vi "test_delay_line_ASIC.vi"(4 "Voltages comprobation":dbl[](array[numeric])=[0.05, 0.06, 0.07, 0.08, 0.09, 0.1, 0.2, 0.3, 0.4, 0.5, 0.6, 0.7, 0.8, 0.9, 1.0], 8 "error in":errorcluster, 9 "Cycles Burst":i32=10000, 11 "Instrument VISA in":T1={"AWG VISA"="generadorpulsos", "Oscilloscope  VISA "="Oscilloscope", "Integration Board IP"="172.16.7.43", "connection ID"=refnum, "report out"=refnum, "report file path"=path "D:/CTA/Data_test/ASIC/delay_line_test"}) -> (0 "error out":errorcluster, 3 "Instrument VISA out":T1={"AWG VISA"="81160A", "Oscilloscope  VISA "="DSO80204B", "Integration Board IP"="172.16.7.43", "connection ID"=refnum, "report out"=refnum, "report file path"=path "D:/CTA/LevelTriggerBoardTest/TestsData/sumtrigger_delay/dataruben"})   [LabVIEW 2009]
uses:
  <vilib>/Utility/NIReport.llb/NI_report.lvclass
  <vilib>/Utility/NIReport.llb/HTML/NI_HTML.lvclass
  <instrlib>/Agilent 8000 Series/Public/Configure/Configure Trigger (Edge).vi
  <instrlib>/Agilent 81150/Agilent 81150.lvlib
  <instrlib>/Agilent 8000 Series/Agilent 8000 Series.lvlib
panel:
  out "Waveform Graph 2":dbl[](graph)
  out "Waveform Graph":dbl[](graph)
  out "XY Graph":cluster{"Y":dbl[], "Y":dbl[]}[](graph)
  out "data read value 18":u32
  out "data out serial 18":string
  out "Data to send hex 18":string
  out "Delay value 2":u16(ring) items=["0", "0.25ns", "0.5ns", "0.75ns", "1ns", "1.25ns", "1.5ns", "1.75ns", "2ns", "2.25ns", "2.5ns", "2.75ns", "3ns", "3.25ns", "3.5ns", "3.75ns", "4ns", "4.25ns", "4.5ns", "4.75ns", "5ns", "5.25ns", "5.5ns", "5.75ns", "2ns_b", "2.25ns_b", "2.5ns_b", "2.75ns_b", "3ns_b", "3.25ns_b", "3.5ns_b", "3.75ns_b", ""]
  out "Id out":i32
  out "Value hex":u32
  in  "Oscilloscope?":bool
  in  "Delay Time (s)":dbl=0.5
  in  "channel":i32
  out "report file path":path
  out "Data output":dbl[][](array[numeric])=[[0.05, 0.0, 0.0, 9.0, 0.0, 0.0, 0.0, 0.0, 0.0, 0.0, 0.0, 0.0, 0.0, 0.0, 0.0, 0.0, 0.036000000000000004, 0.0]]
  out "bucle time":u32=10690
  out "read buffer 3":string
  out "appended array":dbl[](array[numeric])
  out "Numeric":i32=79625954
  in  "Save NOW!":bool
  in  "End 2":bool
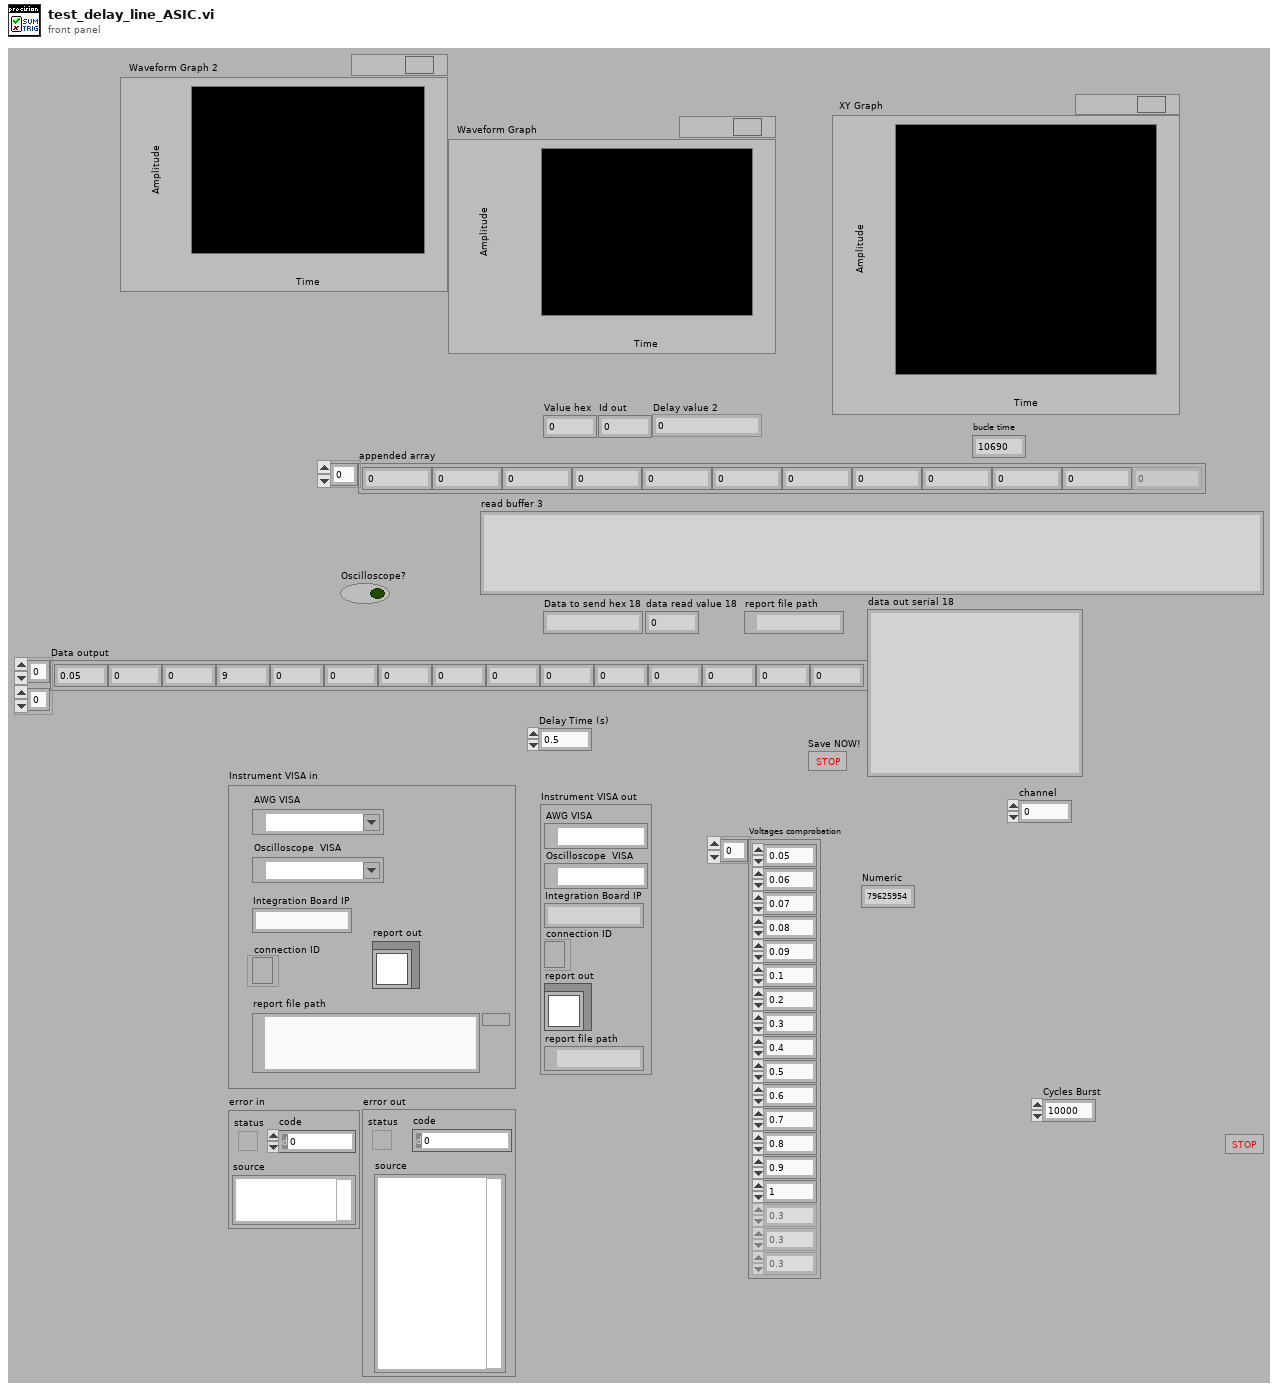
[diagram p1: front panel]
types:
  T1 = cluster{"AWG VISA":refnum<visa-resource-name>, "Oscilloscope  VISA ":refnum<visa-resource-name>, "Integration Board IP":string, "connection ID":refnum<k5>, "report out":refnum<class "NI_report.lvclass">, "report file path":path}
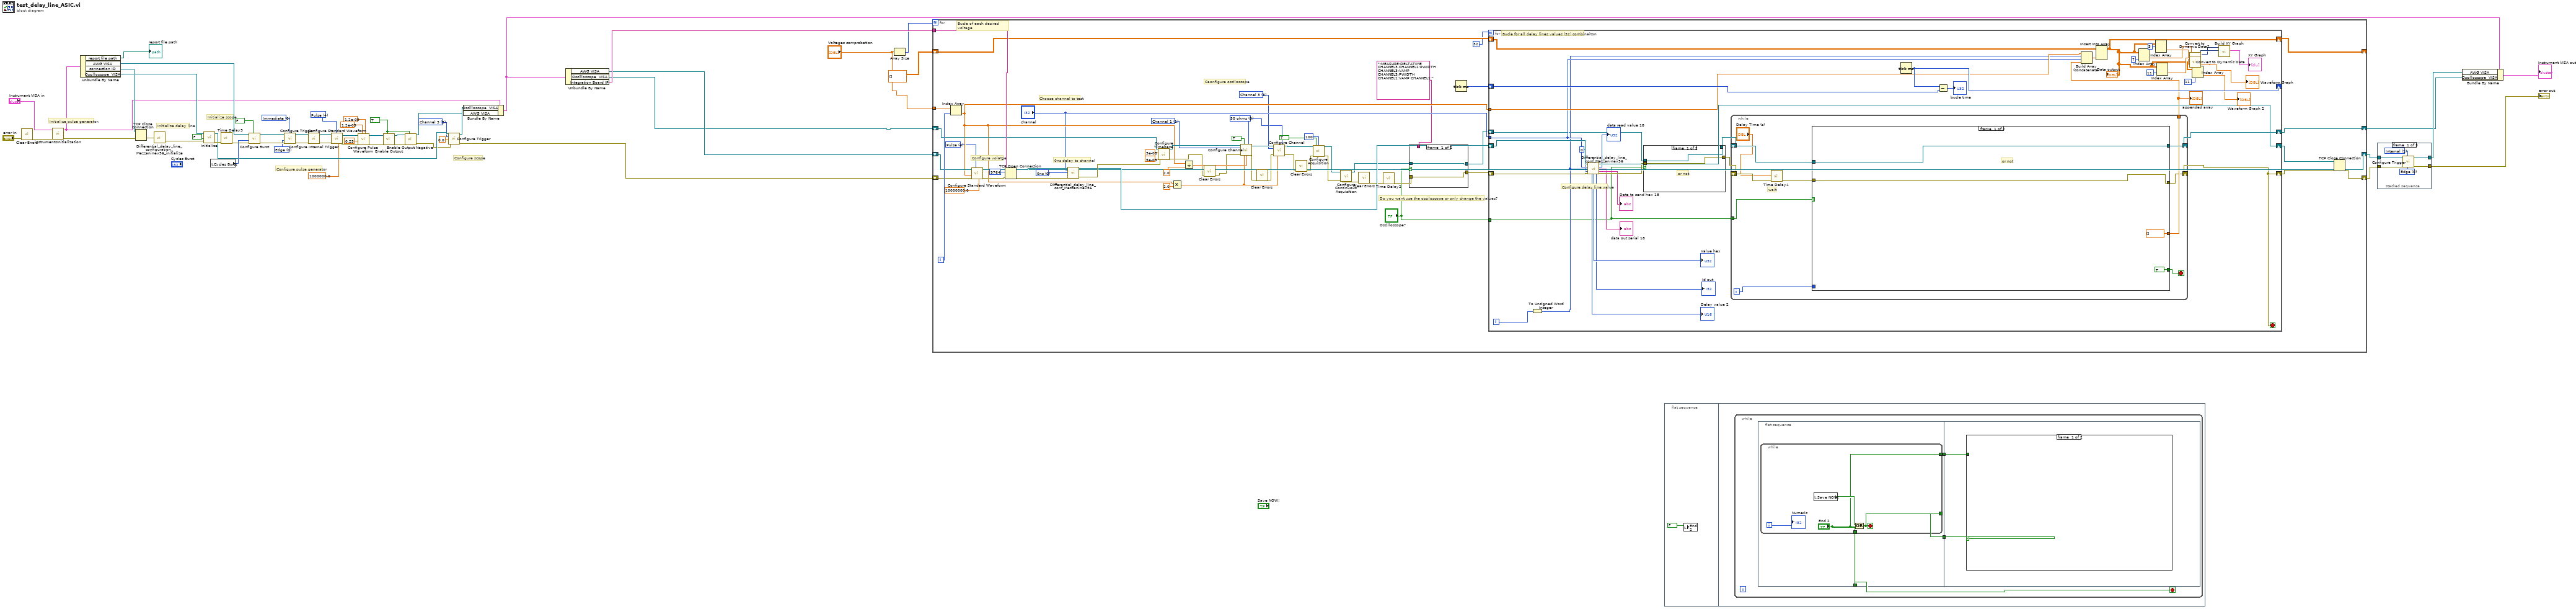
[diagram p0: block diagram]
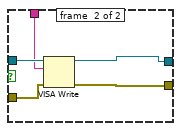
[diagram p2: hidden frame]
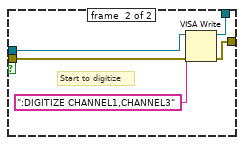
[diagram p3: hidden frame]
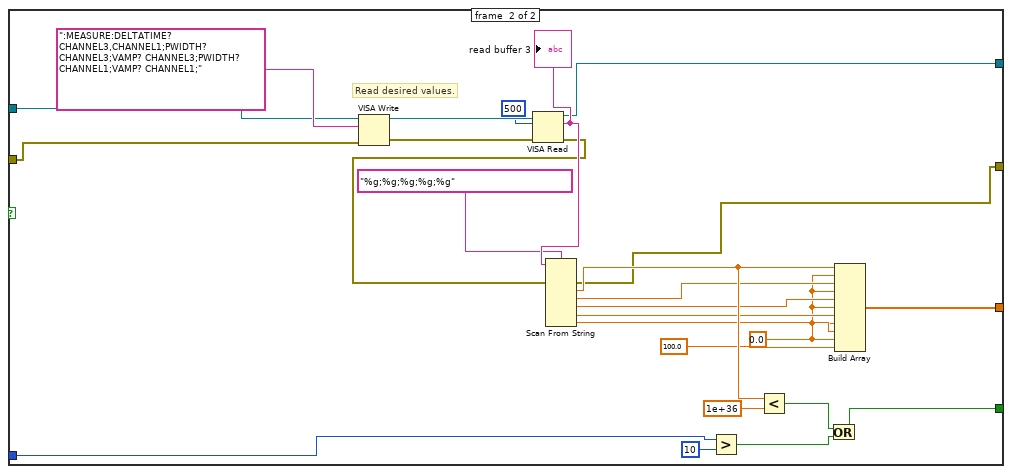
[diagram p4: hidden frame]
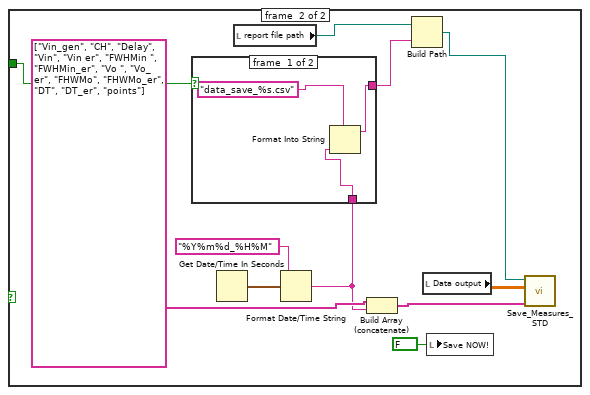
[diagram p5: hidden frame]
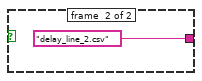
[diagram p6: hidden frame]
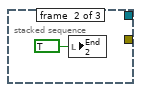
[diagram p7: hidden frame]
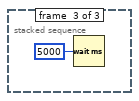
[diagram p8: hidden frame]
diagram:
  w17 = 3 items=["Channel 1"=1, "Channel 2"=2, "Channel 3"=3, "Channel 4"=4, "Digital 0"=13, "Digital 1"=14, "Digital 2"=15, "Digital 3"=16, "Digital 4"=17, "Digital 5"=18, "Digital 6"=19, "Digital 7"=20, "Digital 8"=21, "Digital 9"=22, "Digital 10"=23, "Digital 11"=24, "Digital 12"=25, "Digital 13"=26, "Digital 14"=27, "Digital 15"=28, "Aux"=29, "Line"=30] ("Trigger Source (1: Channel 1)")
  w46 = u16 0 items=["Immediate", "Internal", "External", "Software Trigger Function"] ("Trigger Source (0: Immediate)")
  w47 = u16 0 items=["Edge", "Level"] ("Trigger Mode (0: Edge)")
  w3 = TRUE ("Enable Output (T: Enable)")
  w51 = u16 4 items=["Sine", "Square", "Ramp Up", "Ramp Down", "Pulse", "Noise", "DC"] ("Waveform (0: Sine)")
  # "Configure scope"
  # "Initialize scope"
  # "Configure pulse generator"
  # "Initialize pulse generator."
  # "Initialize delay line"
  n1 = call <vilib>:"Clear Errors.vi"("error in (no error)"="error in") -> ("error out"=w53:errorcluster)  [unwired: 6 in]
  n2 = call "instrumentsInitialization.vi"("error in"=w53, "Instrument VISA in"="Instrument VISA in") -> ("error out"=w21:errorcluster, "Instrument VISA out"=w35:T1)  [unwired: 8 in]
  n3 = Unbundle By Name(w35) -> ("report file path"=→"report file path":path, "AWG VISA"=w37:refnum<visa-resource-name>, "connection ID"=w41:refnum<k5>, "Oscilloscope  VISA"=w38:refnum<visa-resource-name>)
  n4 = TCP Close Connection(connection ID=w41, error in (no error)=w21) -> (error out=w20:errorcluster)  [unwired: 1 in, 1 out]
  n5 = call "Differential_delay_line_configuration_Mezzaninev56_initialize.vi"("error in (no error)"=w20) -> ("error out 2"=w2:errorcluster)  [unwired: 1 in]
  n6 = call <instrlib>:"Initialize.vi"("error in (no error)"=w2, "Reset (True)"=FALSE ("ID Query (True)"), "VISA resource name"=w38) -> ("error out"=w54:errorcluster, "VISA resource name out"=w19:refnum<visa-resource-name>)  [unwired: 7 in]
  n7 = local read "Cycles Burst"() -> (w50:i32)
  n8 = call "Time Delay3"("error in (no error)"=w54) -> ("error out"=w36:errorcluster)  [unwired: 10 in]
  n9 = call <instrlib>:"Configure Burst.vi"("Enable Burst (F: Disable)"=FALSE, "error in (no error)"=w36, "Burst Count (2)"=w50, "VISA resource name"=w37) -> ("error out"=w49:errorcluster, "VISA resource name out"=w48:refnum<visa-resource-name>)  [unwired: 6 in]
  n10 = call <instrlib>:"Configure Trigger.vi"("Trigger Source (0: Immediate)"=w46, "error in (no error)"=w49, "Trigger Mode (0: Edge)"=w47, "VISA resource name"=w48) -> ("error out"=w45:errorcluster, "VISA resource name out"=w44:refnum<visa-resource-name>)  [unwired: 6 in]
  n11 = call <instrlib>:"Configure Internal Trigger.vi"("error in (no error)"=w45, "VISA resource name"=w44) -> ("error out"=w42:errorcluster, "VISA resource name out"=w43:refnum<visa-resource-name>)  [unwired: 8 in]
  n12 = call <instrlib>:"Configure Standard Waveform.vi"("Frequency (1000.0 Hz)"=1000000.0, "Waveform (0: Sine)"=w51, "error in (no error)"=w42, "VISA resource name"=w43) -> ("error out"=w15:errorcluster, "VISA resource name out"=w14:refnum<visa-resource-name>)  [unwired: 6 in]
  n13 = call <instrlib>:"Configure Pulse Waveform.vi"("Trailing Edge Time (7.5E-9 Seconds)"=1.2e-09, "Leading Edge Time (7.5E-9 Seconds)"=1.2e-09, "error in (no error)"=w15, "Duty Cycle (50.0 %)"=0.25, "VISA resource name"=w14) -> ("error out"=w8:errorcluster, "VISA resource name out"=w9:refnum<visa-resource-name>)  [unwired: 5 in]
  n14 = call <instrlib>:"Enable Output.vi"("Enable Output (T: Enable)"=w3, "error in (no error)"=w8, "VISA resource name"=w9) -> ("error out"=w6:errorcluster, "VISA resource name out"=w5:refnum<visa-resource-name>)  [unwired: 7 in]
  n15 = call <instrlib>:"Enable Output Negative.vi"("Enable Output (T: Enable)"=w3, "error in (no error)"=w6, "VISA resource name"=w5) -> ("error out"=w7:errorcluster, "VISA resource name out"=w4:refnum<visa-resource-name>)  [unwired: 7 in]
  n16 = call-poly <instrlib>:"Configure Trigger.vi"("VISA resource name"=w19, "Trigger Source (1: Channel 1)"=w17, "Trigger Level (0.0 V)"=0.0, "error in (no error)"=w7) -> ("VISA resource name out"=w18:refnum<visa-resource-name>, "error out"=w24:errorcluster)  [unwired: 10 in]
  n17 = Bundle By Name(cluster=w35, "Oscilloscope  VISA"=w18, "AWG VISA"=w4) -> (w28:T1)
  n18 = Unbundle By Name(w28) -> ("AWG VISA"=w31:refnum<visa-resource-name>, "Oscilloscope  VISA"=w23:refnum<visa-resource-name>, "Integration Board IP"=w32:string)
  n19 = Array Size(array="Voltages comprobation") -> (size(s)=w27:i32)
  n20 = for {
    N: w27 -> [_]
    tunnel: w32 -> [w112]
    tunnel: "Voltages comprobation" -> [w111]
    shift-right: [w100] -> _
    shift-left: dbl[][] [] -> [w101]
    shift-right: [w98] -> w25
    shift-left: w23 -> [w96]
    shift-right: [w113] -> w33
    shift-left: w24 -> [w86]
    shift-right: [w87] -> w22
    shift-left: w31 -> [w88]
    i -> [w99]
    w75 = 3 items=["Channel 1"=1, "Channel 2"=2, "Channel 3"=3, "Channel 4"=4] ("Channel (1: Channel 1)")
    w83 = u16 4 items=["Sine", "Square", "Ramp Up", "Ramp Down", "Pulse", "Noise", "DC"] ("Waveform (0: Sine)")
    w91 = u16 0 items=["0ns", "0.25ns", "0.5ns", "0.75ns", "1ns", "1.25ns", "1.5ns", "1.75ns", "2ns", "2.25ns", "2.5ns", "2.75ns", "3ns", "3.25ns", "3.5ns", "3.75ns", "4ns", "4.25ns", "4.5ns", "4.75ns", "5ns", "5.25ns", "5.5ns", "5.75ns", "2ns_b", "2.25ns_b", "2.5ns_b", "2.75ns_b", "3ns_b", "3.25ns_b", "3.5ns_b", "3.75ns_b"] ("Delay value")
    w72 = u32 0 items=["50 ohms", "1 Mohms"] ("Input Impedance (1: 1 Mohms)")
    w106 = 1 items=["Channel 1"=1, "Channel 2"=2, "Channel 3"=3, "Channel 4"=4] ("Channel (1: Channel 1)")
    # "Do you want use the osciloscope or only change the values?"
    # "Caonfigure osciloscope"
    # "0ns delay to channel"
    # "Configure volatge"
    # "Choose channel to test"
    # "Bucle of each desired voltage"
    n21 = Index Array(array=w111, index=w99) -> (element=w84:dbl)
    n22 = call <instrlib>:"Configure Standard Waveform.vi"("Frequency (1000.0 Hz)"=10000000.0, "Waveform (0: Sine)"=w83, "error in (no error)"=w86, "Amplitude (1.0 Vpp)"=w84, "VISA resource name"=w88) -> ("error out"=w85:errorcluster, "VISA resource name out"=w87:refnum<visa-resource-name>)  [unwired: 5 in]
    n23 = TCP Open Connection(address=w112, remote port or service name=u16 9764, error in (no error)=w85) -> (connection ID=w94:refnum<k5>, error out=w93:errorcluster)  [unwired: 2 in]
    n24 = call "Differential_delay_line_conf_Mezzaninev56.vi"("connection ID"=w94, "channel"="channel", "Delay value"=w91, "error in (no error)"=w93) -> ("connection ID out"=w90:refnum<k5>, "error out 2"=w92:errorcluster)  [unwired: 4 in, 6 out]
    n25 = call <instrlib>:"Configure Timebase.vi"("error in (no error)"=w92, "Position (0.0 s)"=5e-09, "Timebase (0.005 s)"=5e-08, "VISA resource name"=w96) -> ("error out"=w58:errorcluster, "VISA resource name out"=w107:refnum<visa-resource-name>)  [unwired: 6 in]
    n26 = Multiply(x=w84, y=2.0) -> (x*y=w74:dbl)
    n27 = Divide(x=w84, y=2.0) -> (x/y=w73:dbl)
    n28 = call <vilib>:"Clear Errors.vi"("error in (no error)"=w58) -> ("error out"=w57:errorcluster)  [unwired: 6 in]
    n29 = call <instrlib>:"Configure Channel.vi"("VISA resource name"=w107, "Enable Channel (Enable)"=TRUE, "Input Impedance (1: 1 Mohms)"=w72, "Channel (1: Channel 1)"=w106, "error in (no error)"=w57, "Vertical Range (2.0 V)"=w74, "Vertical Offset (0.0 V)"=w73) -> ("VISA resource name out"=w76:refnum<visa-resource-name>, "error out"=w60:errorcluster)  [unwired: 7 in]
    n30 = call <vilib>:"Clear Errors.vi"("error in (no error)"=w60) -> ("error out"=w59:errorcluster)  [unwired: 6 in]
    n31 = call <instrlib>:"Configure Channel.vi"("VISA resource name"=w76, "Input Impedance (1: 1 Mohms)"=w72, "Channel (1: Channel 1)"=w75, "error in (no error)"=w59, "Vertical Range (2.0 V)"=w74) -> ("VISA resource name out"=w77:refnum<visa-resource-name>, "error out"=w62:errorcluster)  [unwired: 9 in]
    n32 = call <vilib>:"Clear Errors.vi"("error in (no error)"=w62) -> ("error out"=w61:errorcluster)  [unwired: 6 in]
    n33 = call <instrlib>:"Configure Acquisition.vi"("VISA resource name"=w77, "Enable Analog Averaging (Disable)"=TRUE, "Number Of Averages (8)"=100, "error in (no error)"=w61) -> ("VISA resource name out"=w79:refnum<visa-resource-name>, "error out"=w80:errorcluster)  [unwired: 10 in]
    n34 = call <instrlib>:"Configure Continuous Acquisition.vi"("error in (no error)"=w80, "VISA resource name"=w79) -> ("error out"=w64:errorcluster, "VISA resource name out"=w69:refnum<visa-resource-name>)  [unwired: 8 in]
    n35 = call <vilib>:"Clear Errors.vi"("error in (no error)"=w64) -> ("error out"=w63:errorcluster)  [unwired: 6 in]
    n36 = call "Time Delay2"("error in (no error)"=w63) -> ("error out"=w71:errorcluster)  [unwired: 10 in]
    n37 = case shown="True" "Oscilloscope?" {
      tunnel: w71 -> [w114 w120]
      tunnel: [w115 w117] -> w68
      tunnel: w69 -> [w115 w119]
      tunnel: ":MEASURE:DELTATIME CHANNEL3,CHANNEL1;PWIDTH CHANNEL3;VAMP CHANNEL3;PWIDTH CHANNEL1;VAMP CHANNEL1;" ("write buffer") -> [_ w118]
      tunnel: [w114 w116] -> w70
      frame #0 {
      }
      frame #1 {
        n38 = VISA Write(VISA resource name=w119, write buffer=w118, error in (no error)=w120) -> (VISA resource name out=w117:refnum<visa-resource-name>, error out=w116:errorcluster)  [unwired: 1 out]
      }
    }
    n39 = Tick Count (ms)() -> (millisecond timer value=w102:u32)
    n40 = for {
      N: 32 -> [_]
      shift-right: [w133] -> w97
      shift-left: w70 -> [w135]
      shift-right: [w123] -> w100
      shift-left: w101 -> [w159]
      shift-right: [w156] -> w98
      shift-left: w68 -> [w136]
      shift-right: [w155] -> w89
      shift-left: w90 -> [w153]
      shift-right: [w157] -> _
      shift-left: w102 -> [w158]
      tunnel: w84 -> [w154]
      tunnel: "channel" -> [w152]
      tunnel: "Oscilloscope?" -> [w134]
      i -> [w145]
      stop <- w133 stop-if-true
      # "Bucle for all delay lines values (32) combinaiton"
      # "Configure delay line value"
      n41 = To Unsigned Word Integer(number=w145) -> (unsigned 16bit integer=w144:u16)
      n42 = call "Differential_delay_line_conf_Mezzaninev56.vi"("connection ID"=w153, "channel"=w152, "Delay value"=w144, "Id in"=0, "error in (no error)"=w135) -> ("connection ID out"=w155:refnum<k5>, "data read value 18"=→"data read value 18":u32, "data out serial 18"=→"data out serial 18":string, "Data to send hex 18"=→"Data to send hex 18":string, "Delay value out"=→"Delay value 2":u16, "Value hex"=→"Value hex":u32, "Id out"=→"Id out":i32, "error out 2"=w146:errorcluster)  [unwired: 3 in]
      n43 = case shown="True" w134 {
        tunnel: w136 -> [w161 w166]
        tunnel: [w161 w165] -> w148
        tunnel: [w160 w163] -> w147
        tunnel: w146 -> [w160 w162]
        frame #0 {
          # "or not"
        }
        frame #1 {
          # "Start to digitize"
          n44 = VISA Write(VISA resource name=w166, write buffer=":DIGITIZE CHANNEL1,CHANNEL3", error in (no error)=w162) -> (VISA resource name out=w165:refnum<visa-resource-name>, error out=w163:errorcluster)  [unwired: 1 out]
        }
      }
      n45 = while {
        tunnel: [w175] -> w149
        shift-right: [w176] -> w156
        shift-left: w148 -> [w174]
        tunnel: w134 -> [w168]
        shift-right: [w167] -> w133
        shift-left: w147 -> [w170]
        i -> [w173]
        stop <- w172 stop-if-true
        # "wait"
        n46 = call "Time Delay4"("error in (no error)"=w170, "Delay Time (s)"="Delay Time (s)") -> ("error out"=w171:errorcluster)  [unwired: 9 in]
        n47 = case shown="True" w168 {
          tunnel: [w179 w200] -> w176
          tunnel: [dbl[] [] w199] -> w175
          tunnel: [w180 w182] -> w167
          tunnel: w174 -> [w179 w196]
          tunnel: w171 -> [w180 w190]
          tunnel: w173 -> [_ w193]
          tunnel: [TRUE w192] -> w172
          frame #0 {
            # "or not"
          }
          frame #1 {
            w183 = 0.0 ("element")
            # "Read desired values."
            n48 = VISA Write(VISA resource name=w196, write buffer=":MEASURE:DELTATIME? CHANNEL3,CHANNEL1;PWIDTH? CHANNEL3;VAMP? CHANNEL3;PWIDTH? CHANNEL1;VAMP? CHANNEL1;", error in (no error)=w190) -> (VISA resource name out=w205:refnum<visa-resource-name>, error out=w204:errorcluster)  [unwired: 1 out]
            n49 = VISA Read(VISA resource name=w205, byte count=u32 500, error in (no error)=w204) -> (VISA resource name out=w200:refnum<visa-resource-name>, read buffer=w201:string, error out=w197:errorcluster)  [unwired: 1 out]
            "read buffer 3" <- w201
            n50 = Scan From String(format string="%g;%g;%g;%g;%g", input string=w201, error in=w197) -> (error out=w182:errorcluster, output 1=w189:dbl, output 2=w188:dbl, output 3=w187:dbl, output 4=w186:dbl, output 5=w185:dbl)  [unwired: 6 in, 2 out]
            n51 = Greater?(x=w193, y=10) -> (0:w191:bool)
            n52 = Less?(x=w189, y=1e+36) -> (x < y?=w181:bool)
            n53 = Or(x=w181, y=w191) -> (x .or. y?=w192:bool)
            n54 = Build Array(w189, w183, w188, w183, w187, w183, w186, w183, w185, w183, 100.0 ("element")) -> (w199:dbl[])
          }
        }
      }
      "appended array" <- w149
      n55 = Tick Count (ms)() -> (millisecond timer value=w157:u32)
      n56 = Subtract(x=w157, y=w158) -> (x-y=→"bucle time":u32)
      n57 = Build Array (concatenate)(w154, w144, w152, w149) -> (w151:dbl[])
      n58 = Insert Into Array(array=w159, new element=w151) -> (w123:dbl[][])  [unwired: 2 in]
      "Data output" <- w123
      n59 = Index Array(array=w123, index (col)=7 ("disabled index (col)")) -> (element=w127:dbl[])  [unwired: 1 in]
      n60 = Index Array(array=w123, index (col)=3 ("disabled index (col)")) -> (element=→"Waveform Graph":dbl[])  [unwired: 1 in]
      n61 = Index Array(array=w123, index (col)=11 ("disabled index (col)")) -> (element=w129:dbl[])  [unwired: 1 in]
      n62 = call "Convert to Dynamic Data2"("Array"=w127) -> ("Dynamic Data Type"=w126:dynamicdata)  [unwired: 3 in]
      n63 = call "Convert to Dynamic Data"("Array"=w129) -> ("Dynamic Data Type"=w128:dynamicdata)  [unwired: 3 in]
      n64 = Index Array(array=w123, index (col)=11 ("disabled index (col)")) -> (element=→"Waveform Graph 2":dbl[])  [unwired: 1 in]
      n65 = call "Build XY Graph"("Y Input"=w128, "X Input"=w126) -> ("XY Graph"=→"XY Graph":cluster{"Y":dbl[], "Y":dbl[]}[])  [unwired: 8 in, 1 out]
    }
    n66 = TCP Close Connection(connection ID=w89, error in (no error)=w97) -> (error out=w113:errorcluster)  [unwired: 1 in, 1 out]
  }
  n67 = flat-sequence {
    frame #0 {
      n68 = local write "End 2"(FALSE ("End")) -> ()
    }
    frame #1 {
      n69 = while {
        stop <- w207 stop-if-true
        n70 = flat-sequence {
          tunnel: [w212] -> w209
          tunnel: [w211] -> w208
          tunnel: [w210] -> w207
          tunnel: w209 -> [w218]
          tunnel: w208 -> [w217]
          frame #0 {
            n71 = while {
              tunnel: [w215] -> w212
              tunnel: ["End 2"] -> w211
              tunnel: ["End 2"] -> w210
              i -> [w214]
              stop <- w215 stop-if-true
              n72 = local read "Save NOW!"() -> (w216:bool)
              n73 = Or(x=w216, y="End 2") -> (x .or. y?=w215:bool)
              "Numeric" <- w214
            }
          }
          frame #1 {
            n74 = case shown="True" w218 {
              tunnel: w217 -> [_ w226]
              frame #0 {
              }
              frame #1 {
                n75 = Get Date/Time In Seconds() -> (seconds since 1Jan1904=w222:timestamp)
                n76 = local read "report file path"() -> (w228:path)
                n77 = Format Date/Time String(time format string (%c)="%Y%m%d_%H%M", seconds (now)=w222) -> (date/time string=w220:string)  [unwired: 1 in]
                n78 = case shown="True" w226 {
                  tunnel: [w231 "delay_line_2.csv" ("format string")] -> w225
                  tunnel: w220 -> [w230 _]
                  frame #0 {
                    n79 = Format Into String(format string="data_save_%s.csv", w230) -> (resulting string=w231:string)  [unwired: 2 in, 1 out]
                  }
                  frame #1 {
                  }
                }
                n80 = Build Array (concatenate)(string[] ["Vin_gen", "CH", "Delay", "Vin", "Vin er", "FWHMin ", "FWHMin_er", "Vo ", "Vo_er", "FHWMo", "FHWMo_er", "DT", "DT_er", "points"] ("appended array"), w220) -> (w223:string[])
                n81 = Build Path(base path=w228, name or relative path=w225) -> (appended path=w229:path)
                n82 = local read "Data output"() -> (w219:dbl[][])
                n83 = local write "Save NOW!"(FALSE ("Save NOW!")) -> ()
                n84 = call "Save_Measures_STD.vi"("appended array"=w223, "Data in"=w219, "file path (dialog if empty)"=w229) -> ()  [unwired: 9 in]
              }
            }
          }
        }
      }
    }
  }
  n85 = stacked-sequence {
    tunnel: w33 -> [w237 _ _]
    tunnel: [w236 _ _] -> w1
    tunnel: w22 -> [w235 _ _]
    tunnel: [w234 _ _] -> w26
    frame #0 {
      w238 = u16 1 items=["Immediate", "Internal", "External", "Software Trigger Function"] ("Trigger Source (0: Immediate)")
      w239 = u16 0 items=["Edge", "Level"] ("Trigger Mode (0: Edge)")
      n86 = call <instrlib>:"Configure Trigger.vi"("Trigger Source (0: Immediate)"=w238, "error in (no error)"=w237, "Trigger Mode (0: Edge)"=w239, "VISA resource name"=w235) -> ("error out"=w236:errorcluster, "VISA resource name out"=w234:refnum<visa-resource-name>)  [unwired: 6 in]
    }
    frame #1 {
      n87 = local write "End 2"(TRUE ("End 2")) -> ()
    }
    frame #2 {
      n88 = Wait (ms)(milliseconds to wait=u32 5000) -> ()  [unwired: 1 out]
    }
  }
  "error out" <- w1
  n89 = Bundle By Name(cluster=w28, "AWG VISA"=w26, "Oscilloscope  VISA"=w25) -> (→"Instrument VISA out":T1)
